vi "Laser Unit Test.vi"() -> ()   [LabVIEW 2017]
uses:
  builds/Laser.lvlibp/Custom Controls/Command List.ctl
  builds/Laser.lvlibp/Laser.lvclass
  builds/Laser.lvlibp
panel:
  out "Response:":string
  in  "Value":dbl
  in  "Command in":T1=enum."Stop"
  in  "Laser State":bool
  in  "Set PRF":dbl
  in  "Set Power":dbl
  out "PRF":dbl
  out "Output State":bool
  out "Power (mW)":dbl
  in  "Stop":bool
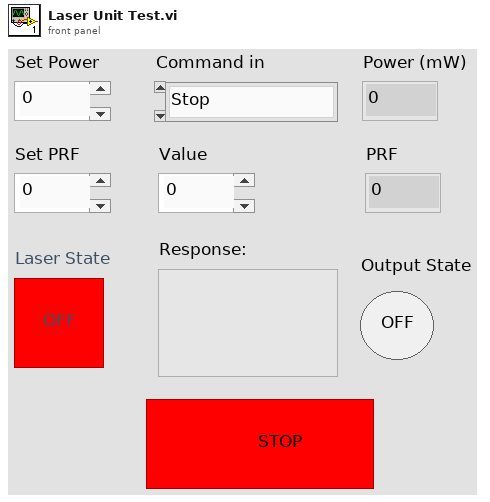
[diagram p1: front panel]
types:
  T1 = typedef "Laser.lvlibp/Command List.ctl" = enum16{"None", "Config?", "Volt?", "ThCase?", "STS?", "Mon?", "Help?", "HB", "Verbose", "Spnt", "Ext", "PRF", "Start", "Stop", "PRF?", "State?", "Status?", "Stat?", "Read HB", "Logon", "Poutmax", "saveconfig", "Reset", "Poutmax?", "PoutCommandMax", "PoutCommandMax?", "FreqMin", "FreqMin?"}
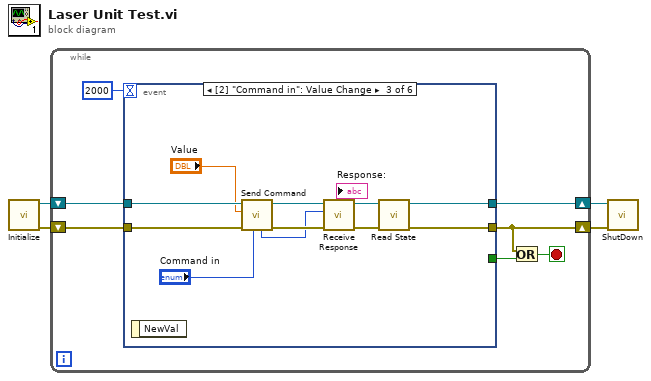
[diagram p0: block diagram]
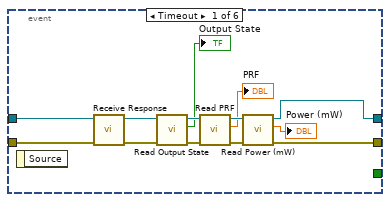
[diagram p2: hidden frame]
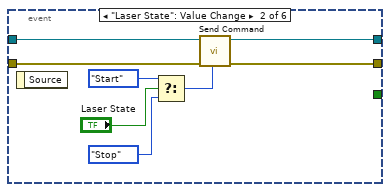
[diagram p3: hidden frame]
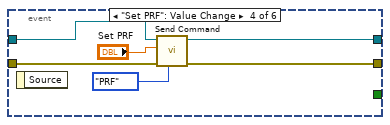
[diagram p4: hidden frame]
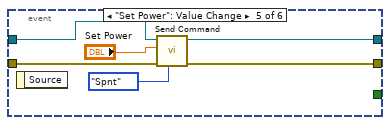
[diagram p5: hidden frame]
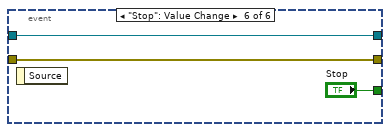
[diagram p6: hidden frame]
diagram:
  n1 = call "Initialize.vi"() -> ("error out"=w3:errorcluster, "Laser out"=w4:refnum<class "Laser.lvclass">)  [unwired: 10 in]
  n2 = while {
    shift-right: [w7] -> w2
    shift-left: w4 -> [w11]
    shift-right: [w6] -> w1
    shift-left: w3 -> [w10]
    stop <- w8 stop-if-true
    n3 = event shown="[2] \"Command in\": Value Change" {
      selector: _ -> [_ _ _ _ _ _]
      dyn-events: _ -> [_ _ _ _ _ _]
      timeout: 2000 -> [_ _ _ _ _ _]
      tunnel: w11 -> [w24 w31 w43 w48 w54 w58]
      tunnel: w10 -> [w23 w32 w42 w49 w55 w57]
      tunnel: [w16 w30 w33 w47 w53 w58] -> w7
      tunnel: [w15 w29 w34 w46 w52 w57] -> w6
      tunnel: [_ _ _ _ _ "Stop"] -> w5
      event Timeout {
        n4 = event-data() -> ()  [unwired: 1 in, 1 out]
        n5 = call-dynamic "Receive Response.vi"("error in (no error)"=w23, "Laser in"=w24) -> ("error out"=w21:errorcluster, "Laser out"=w22:refnum<class "Laser.lvclass">)  [unwired: 8 in]
        n6 = call "Read Output State.vi"("error in (no error)"=w21, "Laser in"=w22) -> ("error out"=w19:errorcluster, "Output State"=→"Output State":bool, "Laser out"=w20:refnum<class "Laser.lvclass">)  [unwired: 7 in]
        n7 = call "Read PRF.vi"("error in (no error)"=w19, "Laser in"=w20) -> ("error out"=w18:errorcluster, "PRF"=→"PRF":dbl, "Laser out"=w17:refnum<class "Laser.lvclass">)  [unwired: 7 in]
        n8 = call "Read Power (mW).vi"("error in (no error)"=w18, "Laser in"=w17) -> ("error out"=w15:errorcluster, "Power (mW)"=→"Power (mW)":dbl, "Laser out"=w16:refnum<class "Laser.lvclass">)  [unwired: 7 in]
      }
      event "Laser State": Value Change {
        n9 = event-data() -> ()  [unwired: 1 in, 1 out]
        n10 = Select(t=Command_List."Start" ("Command in"), s="Laser State", f=Command_List."Stop" ("Command in")) -> (s? t:f=w26:T1)
        n11 = call-dynamic "Send Command.vi"("Command in"=w26, "error in (no error)"=w32, "Laser in"=w31) -> ("error out"=w29:errorcluster, "Laser out"=w30:refnum<class "Laser.lvclass">)  [unwired: 6 in, 1 out]
      }
      event Value Change {
        n12 = event-data() -> ()  [unwired: 1 in, 1 out]
        n13 = call-dynamic "Send Command.vi"("Command in"="Command in", "error in (no error)"=w42, "Value"="Value", "Laser in"=w43) -> ("error out"=w39:errorcluster, "Laser out"=w38:refnum<class "Laser.lvclass">, "Command out"=w37:T1)  [unwired: 5 in]
        n14 = call-dynamic "Receive Response.vi"("error in (no error)"=w39, "Command in"=w37, "Laser in"=w38) -> ("error out"=w36:errorcluster, "Laser out"=w35:refnum<class "Laser.lvclass">)  [unwired: 7 in]
        n15 = call "Read State.vi"("error in (no error)"=w36, "Laser in"=w35) -> ("error out"=w34:errorcluster, "Laser out"=w33:refnum<class "Laser.lvclass">)  [unwired: 7 in, 1 out]
      }
      event "Set PRF": Value Change {
        n16 = event-data() -> ()  [unwired: 1 in, 1 out]
        n17 = call-dynamic "Send Command.vi"("Command in"=Command_List."PRF", "error in (no error)"=w49, "Value"="Set PRF", "Laser in"=w48) -> ("error out"=w46:errorcluster, "Laser out"=w47:refnum<class "Laser.lvclass">)  [unwired: 5 in, 1 out]
      }
      event "Set Power": Value Change {
        n18 = event-data() -> ()  [unwired: 1 in, 1 out]
        n19 = call-dynamic "Send Command.vi"("Command in"=Command_List."Spnt", "error in (no error)"=w55, "Value"="Set Power", "Laser in"=w54) -> ("error out"=w52:errorcluster, "Laser out"=w53:refnum<class "Laser.lvclass">)  [unwired: 5 in, 1 out]
      }
      event "Stop": Value Change {
        n20 = event-data() -> ()  [unwired: 1 in, 1 out]
      }
    }
    n21 = Or(x=w6, y=w5) -> (x .or. y?=w8:bool)
  }
  n22 = call "ShutDown.vi"("error in"=w1, "Laser in"=w2) -> ()  [unwired: 8 in, 2 out]
